vi "Calculate XY From Error.vi"(10 "dt":dbl, 11 "Target Wall Distance":dbl) -> (2 "y":dbl, 3 "x":dbl)   [LabVIEW 2017]
uses:
  Globals/Pose.vi
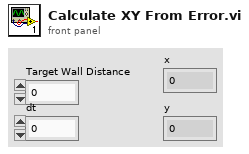
[diagram p1: front panel]
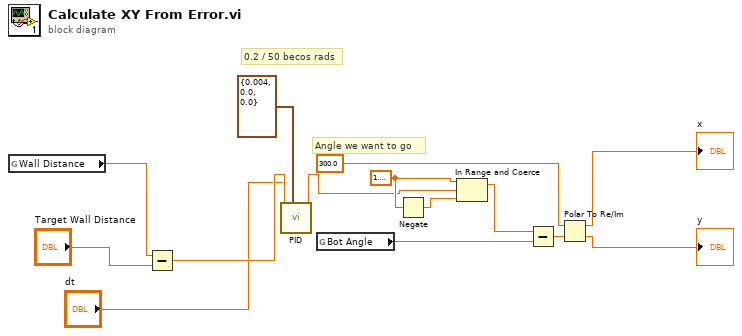
[diagram p0: block diagram]
diagram:
  w4 = 1.5707963267948966
  # "Angle we want to go"
  # "0.2 / 50 becos rads"
  n1 = global read "Pose.vi" "Wall Distance"() -> (w14:dbl)
  n2 = Subtract(x=w14, y="Target Wall Distance") -> (x-y=w12:dbl)
  n3 = call "PID.vi"("PID Gains"=cluster{"P":dbl, "I":dbl, "D":dbl} {"P"=0.004, "I"=0.0, "D"=0.0}, "dt"="dt", "Error"=w12) -> ("result"=w2:dbl)  [unwired: 8 in]
  n4 = global read "Pose.vi" "Bot Angle"() -> (w6:dbl)
  n5 = Negate(x=w4) -> (-x=w3:dbl)
  n6 = In Range and Coerce(upper limit=w4, x=w2, lower limit=w3) -> (coerced(x)=w1:dbl)  [unwired: 1 out]
  n7 = Subtract(x=w1, y=w6) -> (x-y=w5:dbl)
  n8 = Polar To Re/Im(2:w5, 3:300.0 ("r")) -> (0:→"y":dbl, 1:→"x":dbl)
